vi "Get Relay Index.vi"(8 "error in (no error)":errorcluster, 10 "Name":string, 11 "Route Manager in":refnum<class "Route Manager.lvclass">) -> (0 "error out":errorcluster, 2 "Index":i32, 3 "Route Manager out":refnum<class "Route Manager.lvclass">)   [LabVIEW 2015, in "Route Manager.lvclass"]
uses:
  Route Manager.lvclass
  Route Manager.lvclass/Route Manager.ctl
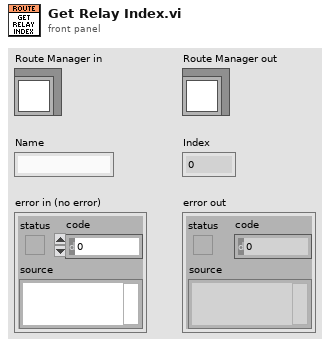
[diagram p1: front panel]
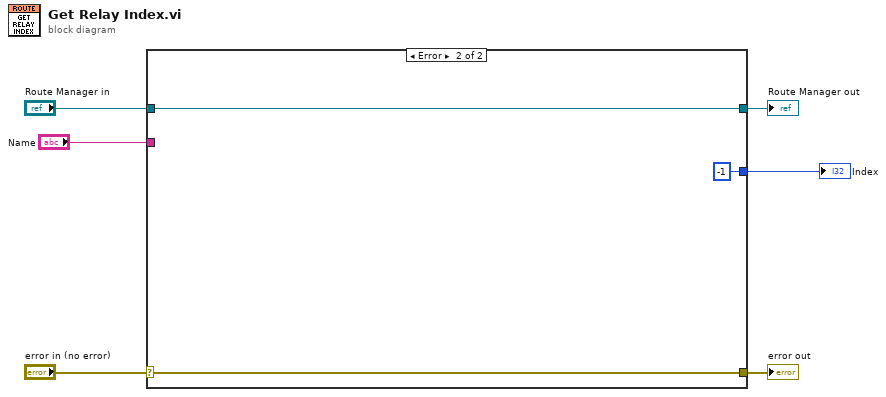
[diagram p0: block diagram]
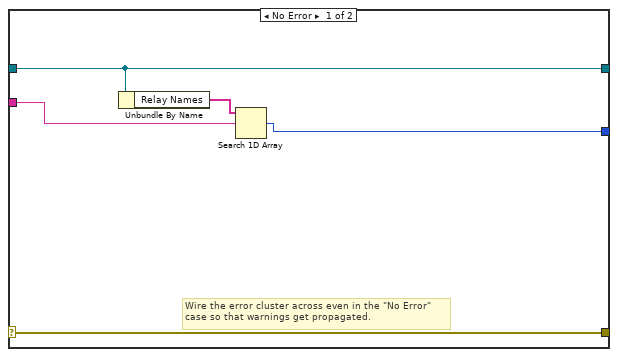
[diagram p2: hidden frame]
diagram:
  n1 = case shown="Error" "error in (no error)" {
    selector: "error in (no error)" -> [w11 w14]
    tunnel: [w11 w14] -> w5
    tunnel: [w10 w13] -> w3
    tunnel: "Route Manager in" -> [w10 w13]
    tunnel: "Name" -> [w8 _]
    tunnel: [w7 -1 ("index of element")] -> w1
    frame No Error {
      # "Wire the error cluster across even in the \"No Error\"\ncase so that warnings get propagated."
      n2 = Unbundle By Name(w10) -> ("Relay Names"=w9:string[])
      n3 = Search 1D Array(1D array=w9, element=w8) -> (index of element=w7:i32)  [unwired: 1 in]
    }
    frame Error {
    }
  }
  "error out" <- w5
  "Route Manager out" <- w3
  "Index" <- w1
